vi "Launcher - Controller.vi"(6 "Worker Alias":string="Controller", 8 "error in":errorcluster, 9 "Initialization Data":T1, 11 "Controller in":refnum<class "Controller.lvclass">) -> (0 "error out":errorcluster)   [LabVIEW 2024]
doc: "This VI launches the Head Worker of a Workers application."
uses:
  Workers/Controller/Initialization Data.ctl
  Workers/Controller/Response Cases.ctl
  <vilib>/addons/_Workers/Library/Case Label.ctl
  Workers/Controller/Controller.lvclass
  C:/Program Files (x86)/National Instruments/LabVIEW 2024/vi.lib/addons/_Workers/Library/Classes/Worker/Worker.lvclass
  <vilib>/addons/_Workers/Debugger/Debug Client/Debug Client.lvlib
  C:/Program Files (x86)/National Instruments/LabVIEW 2024/vi.lib/addons/_Workers/Library/Classes/Workers Object/Workers Object.lvclass
  C:/_Repo/ugm24-dp2/src/Workers/Controller/Controller.lvclass
  <vilib>/addons/_Workers/Library/Workers.lvlib
panel:
  in  "Show Frontpanel":bool
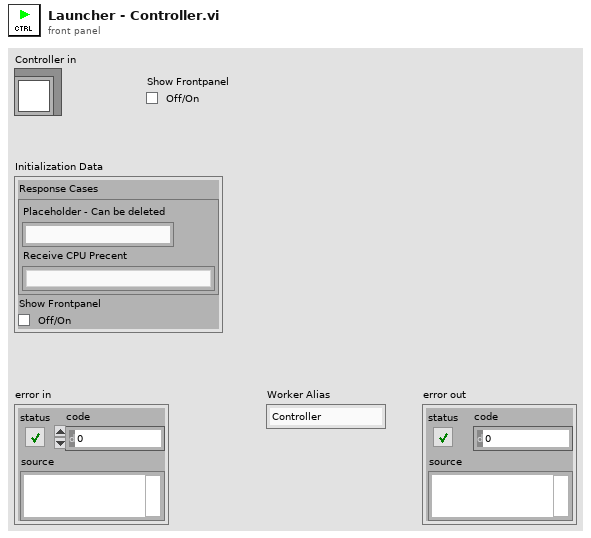
[diagram p1: front panel]
types:
  T1 = typedef "Controller.lvclass/Initialization Data.ctl" = cluster{"Response Cases":T2, "Show Frontpanel":bool}
  T2 = typedef "Controller.lvclass/Response Cases.ctl" = cluster{"Placeholder - Can be deleted":string, "Receive CPU Precent":T3}
  T3 = typedef "Workers.lvlib/Case Label.ctl" = string
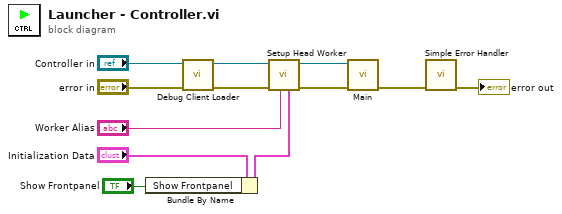
[diagram p0: block diagram]
diagram:
  n1 = Bundle By Name(cluster="Initialization Data", "Show Frontpanel"="Show Frontpanel") -> (w2:T1)
  n2 = call <vilib>:"Debug Client Loader.vi"("error in (no error)"="error in", "Worker_"="Controller in") -> ("error out"=w5:errorcluster, "Worker_out"=w3:refnum<class "Controller.lvclass">)  [unwired: 8 in]
  n3 = call-dynamic "Setup Head Worker.vi"("Initalization Data"=w2, "Worker Alias"="Worker Alias", "error in"=w5, "Worker_"=w3) -> ("error out"=w12:errorcluster, "Worker_out"=w9:refnum<class "Controller.lvclass">)  [unwired: 6 in]
  n4 = call-dynamic "Main.vi"("error in"=w12, "Controller in"=w9) -> ("error out"=w10:errorcluster)  [unwired: 8 in, 1 out]
  n5 = call <vilib>:"Simple Error Handler.vi"("error in (no error)"=w10) -> ("error out"=→"error out":errorcluster)  [unwired: 4 in, 4 out]
